vi "Prevent and Clear Backplane Time Ref Selection.vi"(8 "error in (no error)":errorcluster, 10 "Sync Mod?":bool, 11 "Time Reference Enum":refnum<vi>) -> (0 "error out":errorcluster)   [LabVIEW 2019, in "NI Synchronization System Explorer.lvlib"]
uses:
  NI Synchronization System Explorer.lvlib
  Shared/Time Reference.ctl
  Shared/NI Synchronization Shared.lvlib
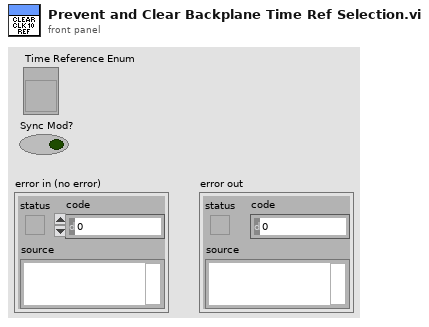
[diagram p1: front panel]
types:
  T1 = typedef "Chassis TimeSync Shared.lvlib/Time Reference.ctl" = enum16{"GPS", "IRIG", "PPS", "1588 Ordinary Clock", "802.1AS", "PXI Chassis Clock", "Free Running (Internal)"}
  T2 = typedef "NI Synchronization Shared.lvlib/Time Reference.ctl" = enum16{"GPS", "IRIG", "PPS", "1588 Ordinary Clock", "802.1AS", "PXI Chassis Clock", "Free Running (Internal)"}
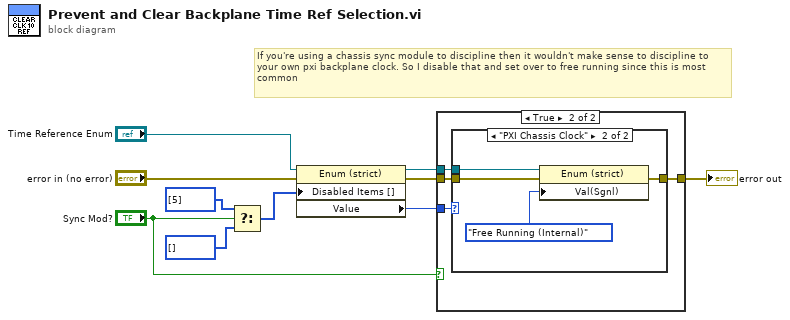
[diagram p0: block diagram]
diagram:
  # "If you're using a chassis sync module to discipline then it wouldn't make sense to discipline to your own pxi backplane clock. So I disable that and set over to free running since this is most common"
  n1 = Select(t=i32[] [5] ("Disabled Items []"), s="Sync Mod?", f=i32[] [] ("Disabled Items []")) -> (s? t:f=w10:i32[])
  n2 = property class="Enum (strict)"(reference="Time Reference Enum", error in="error in (no error)", "Disabled Items []"=w10) -> (reference out=w5:refnum<vi>, error out=w6:errorcluster, "Value"=w2:T1)
  n3 = case shown="True" "Sync Mod?" {
    tunnel: w6 -> [w11 w15]
    tunnel: w5 -> [_ w14]
    tunnel: [w11 w13] -> w4
    tunnel: w2 -> [_ w12]
    frame False {
    }
    frame True {
      n4 = case shown="\"PXI Chassis Clock\"" w12 {
        tunnel: w15 -> [w16 w20]
        tunnel: w14 -> [_ w19]
        tunnel: [w16 w18] -> w13
        frame Default {
        }
        frame "PXI Chassis Clock" {
          n5 = property class="Enum (strict)"(reference=w19, error in=w20, "Val(Sgnl)"=Time_Reference."Free Running (Internal)" ("Value (Signaling)")) -> (error out=w18:errorcluster)  [unwired: 1 out]
        }
      }
    }
  }
  "error out" <- w4
